vi "SingleElementsArray To Data.vi"(7 "Pototype":variant, 8 "error in (no error)":errorcluster, 11 "DataElementArray":variant[](array[variant])) -> (0 "error out":errorcluster, 3 "Cluster":variant)   [LabVIEW 2017]
doc: "Rebuilds a cluster from an array of named elements, using Pototype to supply the target type."
uses:
  <vilib>/Utility/Data Type/Type Definitions/Data Type.ctl
  <vilib>/Utility/Data Type/NI_Data Type.lvlib
  _openG/_reuse_openG.lvlib
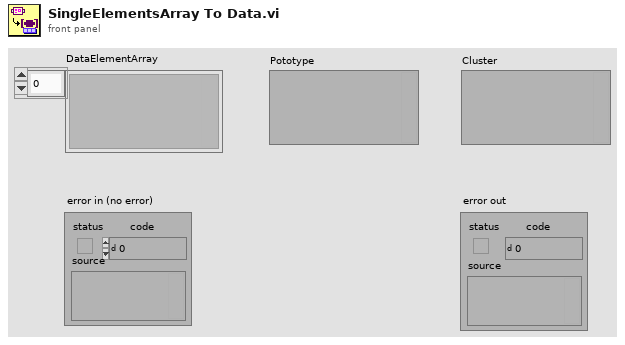
[diagram p1: front panel]
types:
  T1 = typedef "NI_Data Type.lvlib/Data Type.ctl" = enum8{"Invalid Type", "Void", "I8", "I16", "I32", "I64", "U8", "U16", "U32", "U64", "Single Float", "Double Float", "Extended Float", "Single Complex", "Double Complex", "Extended Complex", "Enum U8", "Enum U16", "Enum U32", "Enum U64", "Single Float With Unit", "Double Float With Unit", "Extended Float With Unit", "Single Complex with Unit", "Double Complex with Unit", "Extended Complex with Unit", "Boolean", "String", "Path", "Picture", "Tag", "Array", "Cluster", "Variant", "LV Variant", "Waveform", "Timestamp", "Digital Waveform", "Digital Data", "ExpressData", "Refnum", "External Data", "VI", "Poly VI", "LabVIEW Class Instance", "Fixed Point"}
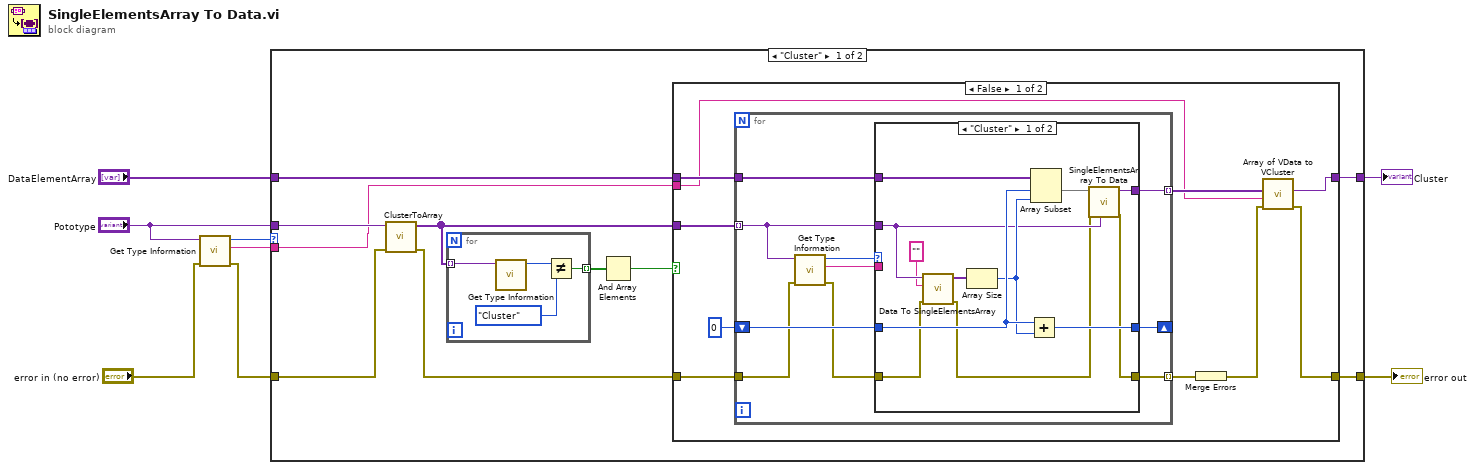
[diagram p0: block diagram]
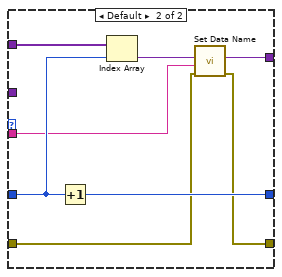
[diagram p2: hidden frame]
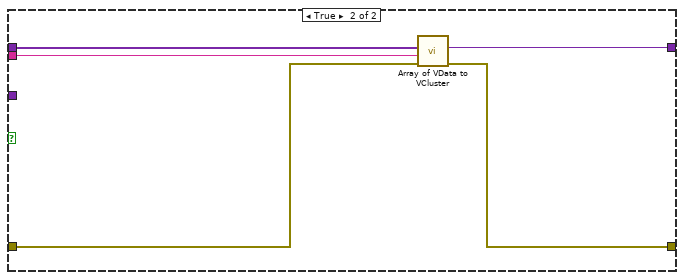
[diagram p3: hidden frame]
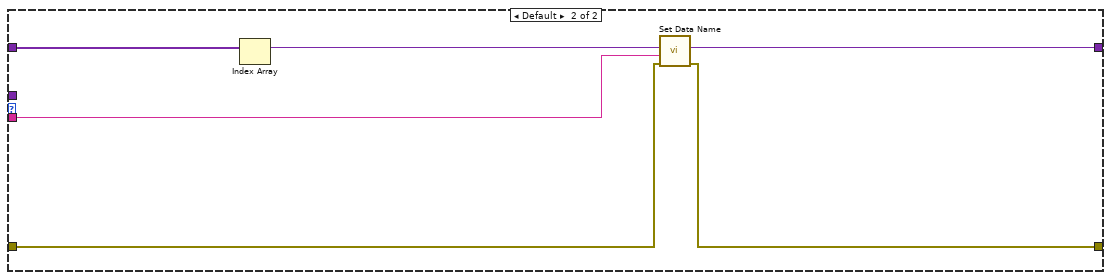
[diagram p4: hidden frame]
diagram:
  n1 = call <vilib>:"Get Type Information.vi"("error in (no error)"="error in (no error)", "Variant"="Pototype") -> ("error out"=w2:errorcluster, "Name"=w1:string, "Type"=w4:T1)  [unwired: 5 in, 2 out]
  n2 = case shown="\"Cluster\"" w4 {
    tunnel: "Pototype" -> [w11 _]
    tunnel: "DataElementArray" -> [w16 w73]
    tunnel: [w15 w71] -> w7
    tunnel: w2 -> [w10 w68]
    tunnel: [w12 w70] -> w6
    tunnel: w1 -> [w9 w69]
    frame "Cluster" {
      n3 = call "ClusterToArray.vi"("Error in"=w10, "Cluster"=w11) -> ("Error out"=w13:errorcluster, "Array"=w14:variant[])  [unwired: 8 in]
      n4 = for {
        tunnel: w14 -> [w66] mode=indexing
        tunnel: [w67] -> w18 mode=indexing
        n5 = call <vilib>:"Get Type Information.vi"("Variant"=w66) -> ("Type"=w65:T1)  [unwired: 6 in, 4 out]
        n6 = Not Equal?(x=w65, y=Data_Type."Cluster") -> (x != y?=w67:bool)
      }
      n7 = And Array Elements(Boolean array=w18) -> (logical AND=w17:bool)
      n8 = case shown="False" w17 {
        tunnel: w16 -> [w24 w63]
        tunnel: [w27 w62] -> w15
        tunnel: w14 -> [w28 _]
        tunnel: w13 -> [w23 w61]
        tunnel: [w19 w60] -> w12
        tunnel: w9 -> [w21 w59]
        frame False {
          n9 = for {
            tunnel: w28 -> [w33] mode=indexing
            tunnel: [w38] -> w26 mode=indexing
            shift-right: [w35] -> _
            shift-left: 0 -> [w36]
            tunnel: w24 -> [w37]
            tunnel: w23 -> [w29]
            tunnel: [w34] -> w22 mode=indexing
            n10 = call <vilib>:"Get Type Information.vi"("error in (no error)"=w29, "Variant"=w33) -> ("error out"=w30:errorcluster, "Name"=w31:string, "Type"=w32:T1)  [unwired: 5 in, 2 out]
            n11 = case shown="\"Cluster\"" w32 {
              tunnel: w33 -> [w44 _]
              tunnel: [w50 w54] -> w38
              tunnel: w37 -> [w49 w58]
              tunnel: w36 -> [w48 w57]
              tunnel: [w46 w56] -> w35
              tunnel: w30 -> [w41 w52]
              tunnel: [w39 w53] -> w34
              tunnel: w31 -> [_ w51]
              frame "Cluster" {
                n12 = call "Data To SingleElementsArray.vi"("error in (no error)"=w41, "parentUrl"="", "Cluster"=w44) -> ("error out"=w40:errorcluster, "DataElementArray"=w42:variant[])  [unwired: 5 in, 2 out]
                n13 = Array Size(array=w42) -> (size(s)=w47:i32)
                n14 = Add(x=w48, y=w47) -> (x+y=w46:i32)
                n15 = Array Subset(array=w49, index=w48, length=w47) -> (w45:variant[])
                n16 = call "SingleElementsArray To Data.vi"("Pototype"=w44, "error in (no error)"=w40, "DataElementArray"=w45) -> ("error out"=w39:errorcluster, "Cluster"=w50:variant)  [unwired: 7 in]
              }
              frame Default {
                n17 = Increment(x=w57) -> (x+1=w56:i32)
                n18 = Index Array(array=w58, index=w57) -> (element=w55:variant)
                n19 = call "Set Data Name.vi"("error in (no error)"=w52, "Data Name"=w51, "Data"=w55) -> ("error out"=w53:errorcluster, "Renamed Data"=w54:variant)  [unwired: 7 in]
              }
            }
          }
          n20 = Merge Errors(w22) -> (w20:errorcluster)
          n21 = call "Array of VData to VCluster.vi"("error in (no error)"=w20, "Cluster Name"=w21, "Array"=w26) -> ("error out"=w19:errorcluster, "VCluster"=w27:variant)  [unwired: 7 in]
        }
        frame True {
          n22 = call "Array of VData to VCluster.vi"("error in (no error)"=w61, "Cluster Name"=w59, "Array"=w63) -> ("error out"=w60:errorcluster, "VCluster"=w62:variant)  [unwired: 7 in]
        }
      }
    }
    frame Default {
      n23 = Index Array(array=w73) -> (element=w72:variant)  [unwired: 1 in]
      n24 = call "Set Data Name.vi"("error in (no error)"=w68, "Data Name"=w69, "Data"=w72) -> ("error out"=w70:errorcluster, "Renamed Data"=w71:variant)  [unwired: 7 in]
    }
  }
  "error out" <- w6
  "Cluster" <- w7
